vi "from string.vi"(8 "error in":errorcluster, 9 "data":string, 10 "version":string, 11 "fixed channel configuration in":refnum<class "fixed channel configuration.lvclass">) -> (0 "error out":errorcluster, 3 "fixed channel configuration out":refnum<class "fixed channel configuration.lvclass">)   [LabVIEW 2013, in "fixed channel configuration.lvclass"]
doc: "Provides an interface for loading a module configuration from a file or other serialized data source. It is recommended that all children of this class store data in two sets--data required for its own initialization, and any data required for parent initialization--and that each implementation uses the <b>Call Parent Method</b> primitive to de-serialize parent information. As a result, it is expected that every module configuration class calls <b>component configuration.lvclass:From String.vi</b>.\nNI Tag Bus Module Framework 1.0.3.43\nNI Systems Engineering"
uses:
  fixed channel configuration.lvclass
  <vilib>/NI/Tag Bus Module Framework/module configuration/TBM module configuration.lvclass
  <vilib>/NI/Tag Bus Module Framework/channel/TBM channel.lvclass
  <vilib>/NI/Configuration Framework/serializable configuration/NISE_CEF_serializable configuration.lvclass
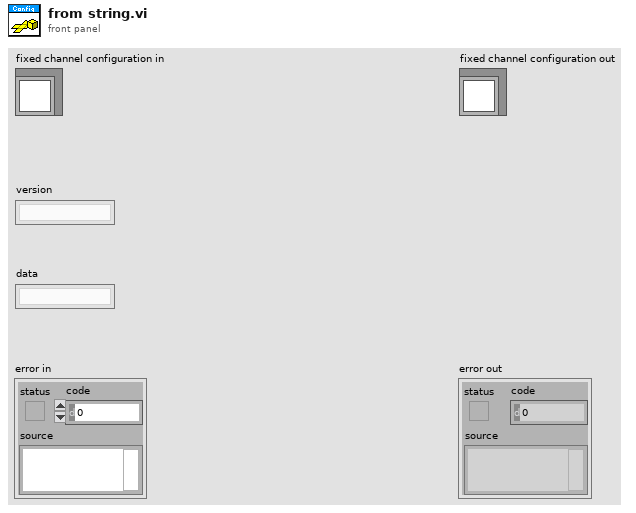
[diagram p1: front panel]
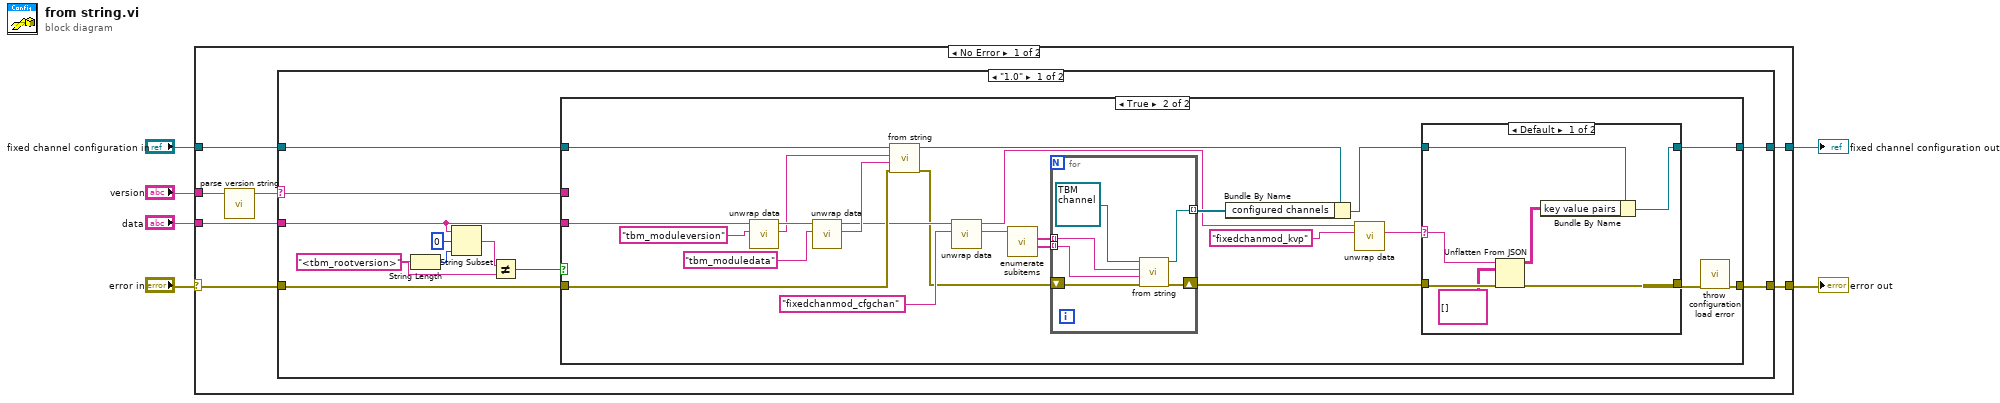
[diagram p0: block diagram]
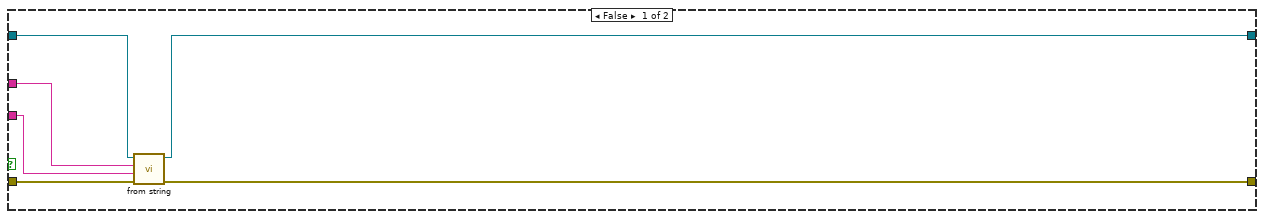
[diagram p2: hidden frame]
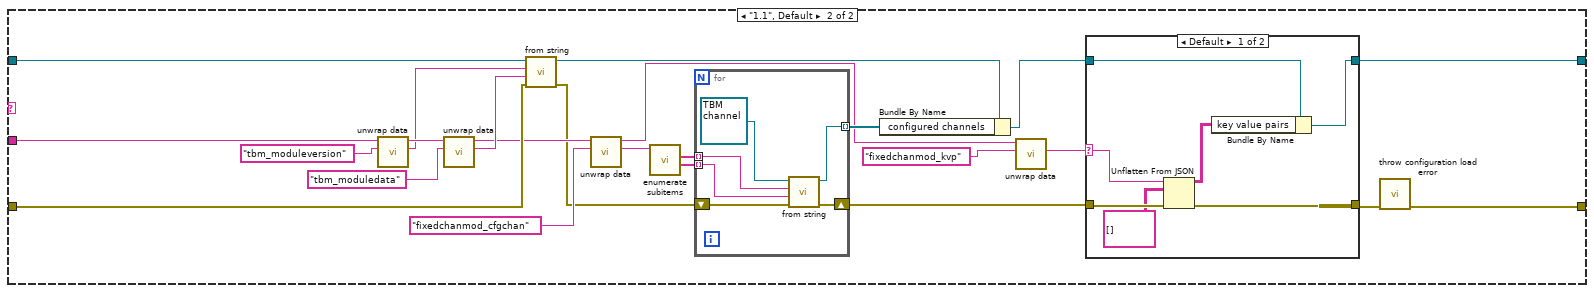
[diagram p4: hidden frame]
diagram:
  n1 = case shown="No Error" "error in" {
    selector: "error in" -> [w7 w110]
    tunnel: "data" -> [w13 _]
    tunnel: "fixed channel configuration in" -> [w12 w109]
    tunnel: [w11 w109] -> w5
    tunnel: [w10 w110] -> w4
    tunnel: "version" -> [w9 _]
    frame No Error {
      n2 = call <vilib>:"parse version string.vi"("full version"=w9) -> ("major.minor version"=w8:string)  [unwired: 7 in, 3 out]
      n3 = case shown="\"1.0\"" w8 {
        selector: w8 -> [w14 _]
        tunnel: w13 -> [w20 w89]
        tunnel: w7 -> [w22 w91]
        tunnel: w12 -> [w24 w93]
        tunnel: [w21 w90] -> w11
        tunnel: [w23 w92] -> w10
        frame "1.0" {
          w18 = "<tbm_rootversion>"
          n4 = String Length(string=w18) -> (length=w19:i32)
          n5 = String Subset(string=w20, offset (0)=0, length (rest)=w19) -> (substring=w17:string)
          n6 = Not Equal?(x=w17, y=w18) -> (x != y?=w16:bool)
          n7 = case shown="True" w16 {
            tunnel: w24 -> [w27 w54]
            tunnel: [w25 w47] -> w23
            tunnel: w22 -> [w30 w46]
            tunnel: [w26 w32] -> w21
            tunnel: w20 -> [w28 w31]
            tunnel: w14 -> [w29 _]
            frame False {
              n8 = call-parent "from string.vi"("error in"=w30, "data"=w28, "version"=w29, "module configuration in"=w27) -> ("error out"=w25:errorcluster, "module configuration out"=w26:refnum<class "fixed channel configuration.lvclass">)  [unwired: 6 in]
            }
            frame True {
              n9 = call <vilib>:"unwrap data.vi"("identifier"="tbm_moduleversion" ("additional identifier"), "data to unwrap"=w31) -> ("unwrapped data"=w48:string, "remaining string"=w50:string)  [unwired: 8 in]
              n10 = call <vilib>:"unwrap data.vi"("identifier"="tbm_moduledata" ("additional identifier"), "data to unwrap"=w50) -> ("unwrapped data"=w49:string, "remaining string"=w44:string)  [unwired: 8 in]
              n11 = call-parent "from string.vi"("error in"=w46, "data"=w49, "version"=w48, "module configuration in"=w54) -> ("error out"=w42:errorcluster, "module configuration out"=w53:refnum<class "fixed channel configuration.lvclass">)  [unwired: 6 in]
              n12 = call <vilib>:"unwrap data.vi"("identifier"="fixedchanmod_cfgchan", "data to unwrap"=w44) -> ("unwrapped data"=w43:string, "remaining string"=w38:string)  [unwired: 8 in]
              n13 = call <vilib>:"enumerate subitems.vi"("data to enumerate"=w43) -> ("associated data"=w40:string[], "discovered subitems"=w41:string[])  [unwired: 8 in, 1 out]
              n14 = for {
                shift-right: [w69] -> w36
                shift-left: w42 -> [w68]
                tunnel: w41 -> [w66] mode=indexing
                tunnel: w40 -> [w65] mode=indexing
                tunnel: [w67] -> w39 mode=indexing
                n15 = call-dynamic "from string.vi"("error in"=w68, "channel data"=w65, "identifier"=w66, "channel in"=refnum<class "TBM channel.lvclass"> refnum) -> ("error out"=w69:errorcluster, "channel out"=w67:refnum<class "TBM channel.lvclass">)  [unwired: 6 in]
              }
              n16 = Bundle By Name(cluster=w53, "configured channels"=w39) -> (w33:refnum<class "fixed channel configuration.lvclass">)
              n17 = call <vilib>:"unwrap data.vi"("identifier"="fixedchanmod_kvp", "data to unwrap"=w38) -> ("unwrapped data"=w35:string)  [unwired: 8 in, 1 out]
              n18 = case shown="Default" w35 {
                selector: w35 -> [w57 _]
                tunnel: w36 -> [w59 w63]
                tunnel: [w58 w63] -> w34
                tunnel: w33 -> [w61 w62]
                tunnel: [w60 w62] -> w32
                frame Default {
                  n19 = Unflatten From JSON(JSON string=w57, type and defaults=string[][] [] ("key value pairs"), error in (no error)=w59) -> (value=w56:string[][], error out=w58:errorcluster)  [unwired: 4 in]
                  n20 = Bundle By Name(cluster=w61, "key value pairs"=w56) -> (w60:refnum<class "fixed channel configuration.lvclass">)
                }
                frame "" {
                }
              }
              n21 = call <vilib>:"throw configuration load error.vi"("error in"=w34) -> ("error out"=w47:errorcluster)  [unwired: 10 in]
            }
          }
        }
        frame "1.1", Default {
          n22 = call <vilib>:"unwrap data.vi"("identifier"="tbm_moduleversion" ("additional identifier"), "data to unwrap"=w89) -> ("unwrapped data"=w83:string, "remaining string"=w85:string)  [unwired: 8 in]
          n23 = call <vilib>:"unwrap data.vi"("identifier"="tbm_moduledata" ("additional identifier"), "data to unwrap"=w85) -> ("unwrapped data"=w84:string, "remaining string"=w81:string)  [unwired: 8 in]
          n24 = call-parent "from string.vi"("error in"=w91, "data"=w84, "version"=w83, "module configuration in"=w93) -> ("error out"=w79:errorcluster, "module configuration out"=w88:refnum<class "fixed channel configuration.lvclass">)  [unwired: 6 in]
          n25 = call <vilib>:"unwrap data.vi"("identifier"="fixedchanmod_cfgchan", "data to unwrap"=w81) -> ("unwrapped data"=w80:string, "remaining string"=w75:string)  [unwired: 8 in]
          n26 = call <vilib>:"enumerate subitems.vi"("data to enumerate"=w80) -> ("associated data"=w77:string[], "discovered subitems"=w78:string[])  [unwired: 8 in, 1 out]
          n27 = for {
            shift-right: [w108] -> w73
            shift-left: w79 -> [w107]
            tunnel: w78 -> [w105] mode=indexing
            tunnel: w77 -> [w104] mode=indexing
            tunnel: [w106] -> w76 mode=indexing
            n28 = call-dynamic "from string.vi"("error in"=w107, "channel data"=w104, "identifier"=w105, "channel in"=refnum<class "TBM channel.lvclass"> refnum) -> ("error out"=w108:errorcluster, "channel out"=w106:refnum<class "TBM channel.lvclass">)  [unwired: 6 in]
          }
          n29 = Bundle By Name(cluster=w88, "configured channels"=w76) -> (w70:refnum<class "fixed channel configuration.lvclass">)
          n30 = call <vilib>:"unwrap data.vi"("identifier"="fixedchanmod_kvp", "data to unwrap"=w75) -> ("unwrapped data"=w72:string)  [unwired: 8 in, 1 out]
          n31 = case shown="Default" w72 {
            selector: w72 -> [w96 _]
            tunnel: w73 -> [w98 w102]
            tunnel: [w97 w102] -> w71
            tunnel: w70 -> [w100 w101]
            tunnel: [w99 w101] -> w90
            frame Default {
              n32 = Unflatten From JSON(JSON string=w96, type and defaults=string[][] [] ("key value pairs"), error in (no error)=w98) -> (value=w95:string[][], error out=w97:errorcluster)  [unwired: 4 in]
              n33 = Bundle By Name(cluster=w100, "key value pairs"=w95) -> (w99:refnum<class "fixed channel configuration.lvclass">)
            }
            frame "" {
            }
          }
          n34 = call <vilib>:"throw configuration load error.vi"("error in"=w71) -> ("error out"=w92:errorcluster)  [unwired: 10 in]
        }
      }
    }
    frame Error {
    }
  }
  "error out" <- w4
  "fixed channel configuration out" <- w5
